vi "onHttpPost (File).vi"(6 "timeout":i32=10000, 7 "output file":path, 8 "error in":errorcluster, 9 "file":path, 10 "url":string, 11 "advanced-http-client in":refnum<class "advanced-http-client.lvclass">) -> (0 "error out":errorcluster, 1 "body":string, 2 "headers":string, 3 "advanced-http-client out":refnum<class "advanced-http-client.lvclass">)   [LabVIEW 2020, in "advanced-http-client.lvclass"]
uses:
  advanced-http-client.lvclass
  advanced-http-client.lvclass/advanced-http-client.ctl
  <vilib>/NI/Advanced HTTP Client/POST (File).vi
  <vilib>/NI/Advanced HTTP Client/Session.lvclass
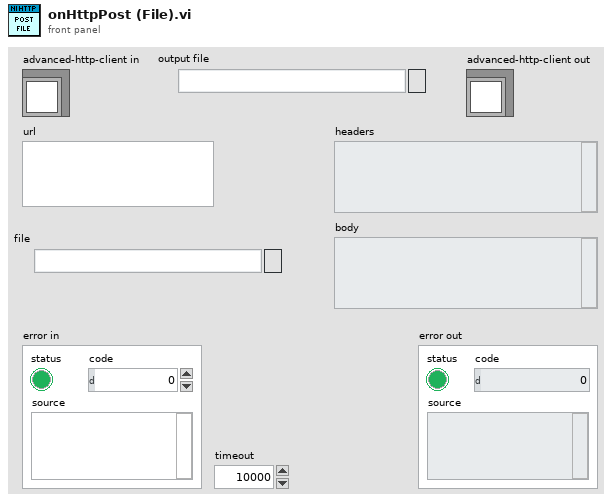
[diagram p1: front panel]
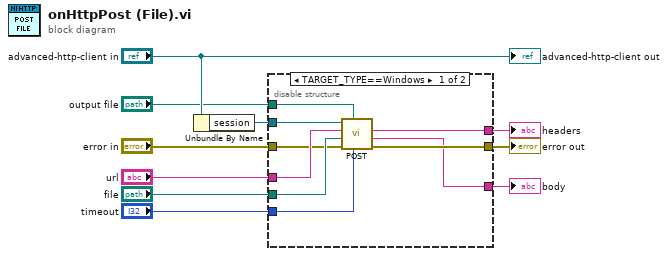
[diagram p0: block diagram]
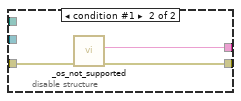
[diagram p2: hidden frame]
diagram:
  n1 = Unbundle By Name("advanced-http-client in") -> ("session"=w9:refnum<class "Session.lvclass">)
  n2 = disable-structure shown="TARGET_TYPE==Windows" {
    disable-tunnel: w9 -> [w19 _]
    disable-tunnel: "output file" -> [w18 _]
    disable-tunnel: "url" -> [w17 _]
    disable-tunnel: "file" -> [w16 _]
    disable-tunnel: "error in" -> [w15 w22]
    disable-tunnel: "timeout" -> [w14 _]
    disable-tunnel: [w13 w21] -> w3
    disable-tunnel: [w12 _] -> w2
    disable-tunnel: [w11 w20] -> w1
    frame condition #0 (active) {
      n3 = call-poly <vilib>:"POST.vi"("timeout"=w14, "output file"=w18, "error in"=w15, "file"=w16, "url"=w17, "session in"=w19) -> ("error out"=w13:errorcluster, "body"=w12:string, "headers"=w11:string)  [unwired: 1 in, 2 out]
    }
    frame condition #1 {
      n4 = call "_os_not_supported.vi"("error in (no error)"=w22) -> ("error out"=w21:errorcluster, "headers"=w20:string)  [unwired: 9 in]
    }
  }
  "error out" <- w3
  "headers" <- w1
  "body" <- w2
  "advanced-http-client out" <- "advanced-http-client in"
